vi "Clear Entire Configuration.vi"(8 "error in (no error)":errorcluster, 11 "Item Ref in":T1 format="%.0x") -> (0 "error out":errorcluster)   [LabVIEW 2015, in "Engine Simulation Toolkit System Explorer.lvlib"]
uses:
  Engine Simulation Toolkit System Explorer.lvlib
  <vilib>/NI Veristand/Custom Device API/Custom Device Item Ref.ctl
  Shared/Properties.vi
  Shared/Constants and GUIDs.vi
  <vilib>/NI Veristand/Custom Device Tools/Custom Device Utility Library/NI VeriStand - Search for All Items by GUID.vi
  <vilib>/NI Veristand/Custom Device API/Custom Device API.lvlib
  Shared/Engine Simulation Toolkit Shared.lvlib
  <vilib>/NI Veristand/Custom Device Tools/Custom Device Utility Library/Custom Device Utility Library.lvlib
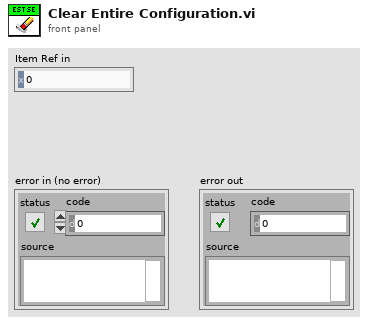
[diagram p1: front panel]
types:
  T1 = typedef "Custom Device API.lvlib/Custom Device Item Ref.ctl" = u64
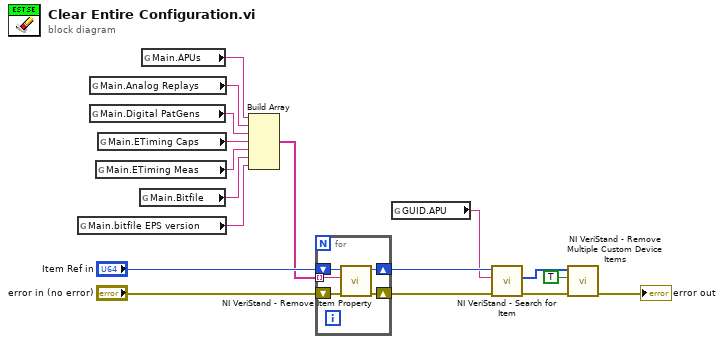
[diagram p0: block diagram]
diagram:
  n1 = global read "Properties.vi" "Main.bitfile EPS version"() -> (w3:string)
  n2 = global read "Properties.vi" "Main.Analog Replays"() -> (w6:string)
  n3 = global read "Properties.vi" "Main.Digital PatGens"() -> (w7:string)
  n4 = global read "Properties.vi" "Main.ETiming Meas"() -> (w9:string)
  n5 = global read "Properties.vi" "Main.ETiming Caps"() -> (w8:string)
  n6 = global read "Properties.vi" "Main.Bitfile"() -> (w4:string)
  n7 = global read "Properties.vi" "Main.APUs"() -> (w5:string)
  n8 = Build Array(w5, w6, w7, w8, w9, w4, w3) -> (w2:string[])
  n9 = for {
    shift-right: [w20] -> w12
    shift-left: "error in (no error)" -> [w22]
    shift-right: [w19] -> w13
    shift-left: "Item Ref in" -> [w21]
    tunnel: w2 -> [w18] mode=indexing
    n10 = call <vilib>:"NI VeriStand - Remove Item Property.vi"("error in (no error)"=w22, "Property Name"=w18, "Item Ref in"=w21) -> ("error out"=w20:errorcluster, "Item Ref out"=w19:T1)  [unwired: 6 in, 1 out]
  }
  n11 = global read "Constants and GUIDs.vi" "GUID.APU"() -> (w1:string)
  n12 = call-poly <vilib>:"NI VeriStand - Search for Item.vi"("error in"=w12, "Item GUID"=w1, "Section Ref in"=w13) -> ("error out"=w14:errorcluster, "Item Refs"=w16:T1[])  [unwired: 5 in, 2 out]
  n13 = call <vilib>:"NI VeriStand - Remove Multiple Custom Device Items.vi"("error in (no error)"=w14, "Force Delete (F)"=TRUE, "Item Refs in"=w16) -> ("error out"=→"error out":errorcluster)  [unwired: 7 in, 1 out]
